vi "Drive Controller.vi"(8 "error in":errorcluster) -> ()   [LabVIEW 2017]
doc: "This VI executes continuously carrying out the current operation and responding to updates or new operation requests. It will often contain the timing or control code that is difficult to place directly in TeleOp. This VI generally opens all sensors and motors and isolates the rest of the robot code from knowing implementation details of how the operations are carried out."
uses:
  <vilib>/Rock Robotics/WPI/Framework/Completion Status.ctl
  Drive Setpoints.ctl
  Drive Operations.ctl
  <vilib>/Rock Robotics/WPI/SafetyOutput/WPI_SafetyOutputConfigMenu.ctl
  Public/Documents/Cross The Road Electronics/Phoenix-LabVIEW/Motor Controller/Controls/CTRE_Phoenix_MotorControl_FeedbackDevice.ctl
  Drive Published Globals.vi
  <vilib>/Rock Robotics/WPI/RobotDrive/WPI_RobotDriveOpen2MotorWithExistingMotors.vi
  Framework/Robot Global Data.vi
  Public/Documents/Cross The Road Electronics/Phoenix-LabVIEW/Motor Controller/Get/CTRE_Phoenix_MotorController_GetQuadratureData.vi
  <vilib>/Rock Robotics/WPI/RobotDrive/WPI_RobotDriveArcadeDrive_Standard(NoSaturation).vi
  <vilib>/Rock Robotics/Network Tables/NT Write Numeric Array.vi
panel:
  out "UseLDriveEncoder":bool
  out "LDriveEncoder":i32
  out "RDriveEncoder":i32
  out "DriveLastCommandStatus":T1
  in  "Interactive Values":T2
  in  "Buttons":cluster{"Execute Cmd":bool, "Abort Cmd":bool}
  out "Command Timing":cluster{"Start Time (ms)":u32, "Iterations":i32}
  out "Status":T1
  out "Setpoints":T4(graph)
  out "Current\nCmd":string
  # "Tip: The graph shows the motor setpoints. It may also be helpful to observe inputs and sensor values.\nYou may also want to display tuning or debugging controls."
  # "Interactive Command: You may fill in the settings for a command\nand schedule it with the Execute button. You can observe and abort\nany command while fine tuning the code for the controller."
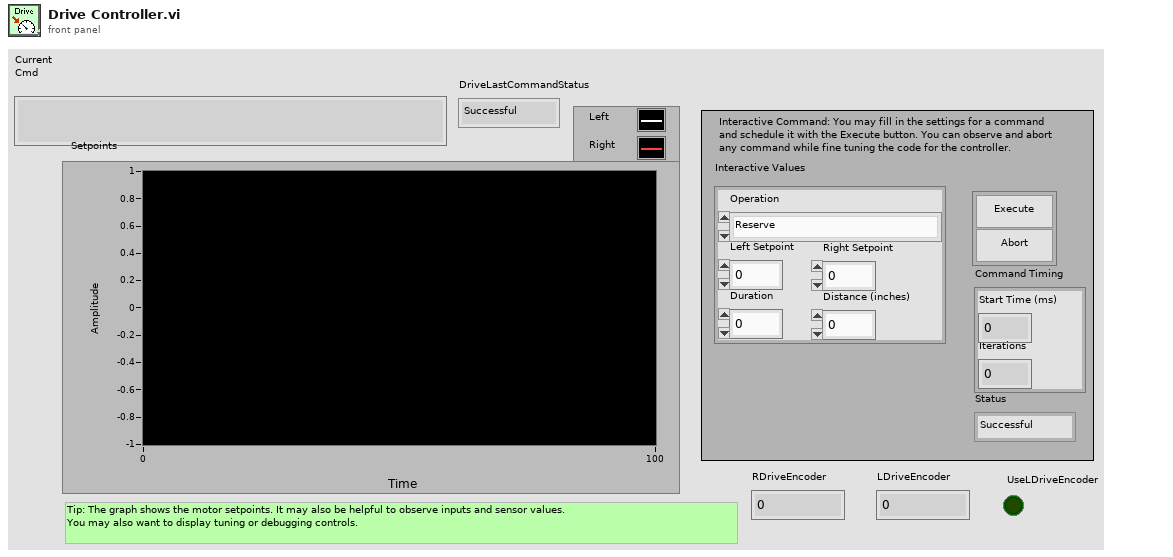
[diagram p1: front panel]
types:
  T1 = typedef "Completion Status.ctl" = enum16{"Successful", "Aborted", "Incomplete"}
  T2 = typedef "Drive Setpoints.ctl" = cluster{"Operation":T3, "Left Setpoint":dbl, "Right Setpoint":dbl, "Duration":dbl, "Distance (inches)":dbl}
  T3 = typedef "Drive Operations.ctl" = enum16{"Reserve", "Read Current", "Immediate", "Drive for Time", "Drive for Distance"}
  T4 = cluster{"Left Setpoint":dbl, "Right Setpoint":dbl}
  T5 = typedef "WPI_SafetyOutputConfigMenu.ctl" = enum16{"Enable", "Disable"}
  T6 = typedef "CTRE_Phoenix_MotorControl_FeedbackDevice.ctl" = i8
  T7 = typedef "WPI_MotorControlDeviceRef.ctl" = cluster{"DeviceStatus":errorcluster, "Type":T8, "PWM":cluster{"PWM Channel":T9, "DeadBand":T10}, "CAN":cluster{"Device Number":u8, "SetOutput VI Ref":variant, "GetOutput VI Ref":variant, "Enable VI Ref":variant, "Disable VI Ref":variant, "Data":variant}, "Invert":bool, "DIO PWM":cluster{"PWM \"Enable\" Channel":T9, "DIOChannel":T11, "PWM Rate":dbl}}
  T8 = typedef "WPI_MotorControlType.ctl" = enum16{"PWM", "CAN", "DIO PWM"}
  T9 = typedef "FPGA_DIOPWMChannel.ctl" = enum8{"PWM 0", "PWM 1", "PWM 2", "PWM 3", "PWM 4", "PWM 5", "PWM 6", "PWM 7", "PWM 8", "PWM 9", "PWM MXP 0", "PWM MXP 1", "PWM MXP 2", "PWM MXP 3", "PWM MXP 4", "PWM MXP 5", "PWM MXP 6", "PWM MXP 7", "PWM MXP 8", "PWM MXP 9", "Invalid"}
  T10 = typedef "WPI_PWMDeadband.ctl" = cluster{"Name":string, "maxPositivePwm":i32, "minPositivePwm":i32, "centerPwm":i32, "maxNegativePwm":i32, "minNegativePwm":i32, "angularRange":u16}
  T11 = typedef "FPGA_DIOChannel.ctl" = enum8{"DIO 0", "DIO 1", "DIO 2", "DIO 3", "DIO 4", "DIO 5", "DIO 6", "DIO 7", "DIO 8", "DIO 9", "DIO MXP 0", "DIO MXP 1", "DIO MXP 2", "DIO MXP 3", "DIO MXP 4", "DIO MXP 5", "DIO MXP 6", "DIO MXP 7", "DIO MXP 8", "DIO MXP 9", "DIO MXP 10", "DIO MXP 11", "DIO MXP 12", "DIO MXP 13", "DIO MXP 14", "DIO MXP 15", "SPI Port CS1", "SPI Port CS2", "SPI Port CS3", "SPI Port MISO", "SPI Port MOSI", "Invalid"}
  T12 = typedef "WPI_RobotDriveDevRef.ctl" = cluster{"DevStatus":errorcluster, "Motors[]":T7[], "Square Inputs":bool, "Max Output":dbl}
  T13 = typedef "Command Status Info.ctl" = cluster{"Name":string, "Status":T1, "notifier out":T14}
  T14 = typedef "Completion Notifier.ctl" = refnum<notifier>
  T15 = cluster{"SubSystem Data":T2, cluster{"Start Time (ms)":u32, "Iterations":i32}, cluster{"Command Info":T13, "Description":string, "Default Command":T2, "queue out":refnum<queue>, "Subsystem Name":string}}
  T16 = cluster{"SubSystem Data":T2, cluster{"Start Time (ms)":u32, "Iterations":i32}, "Default Command Arguments":cluster{"Command Info":T13, "Description":string, "Default Command":T2, "queue out":refnum<queue>, "Subsystem Name":string}}
  T17 = cluster{"Don't move motors while reserved":dbl, "Don't move motors while reserved":dbl}
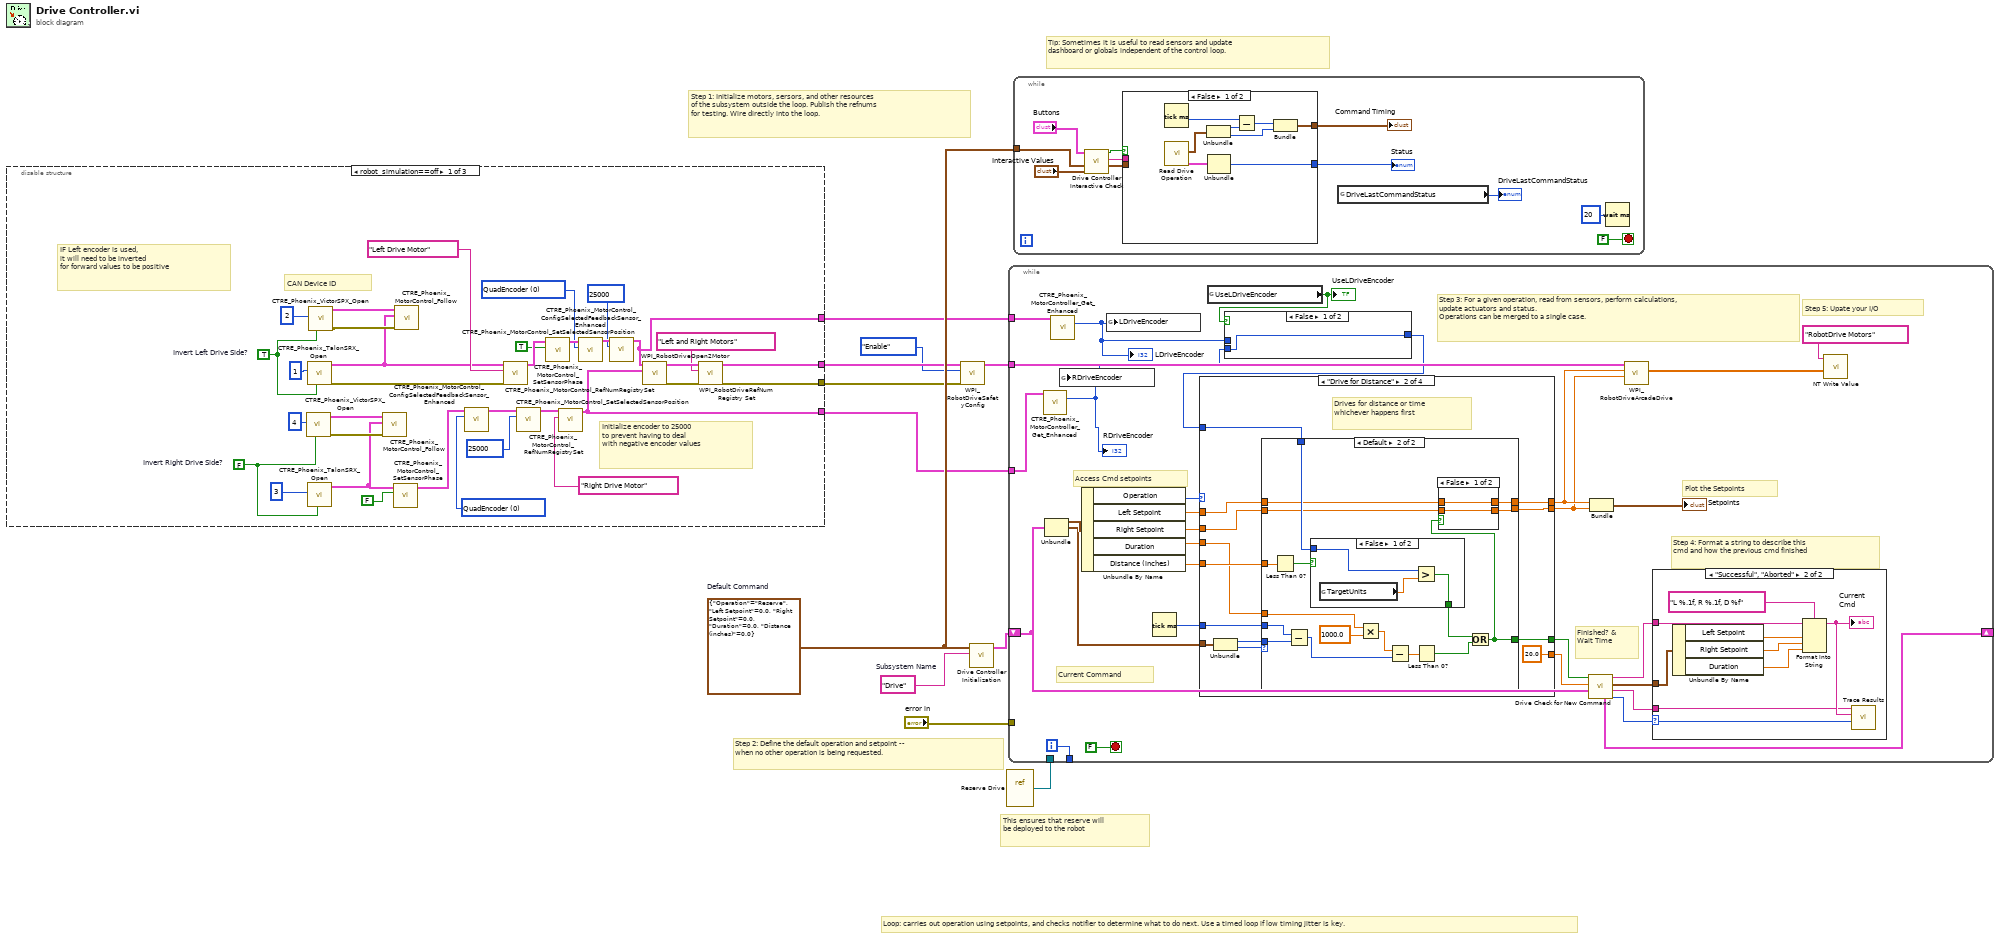
[diagram p0: block diagram]
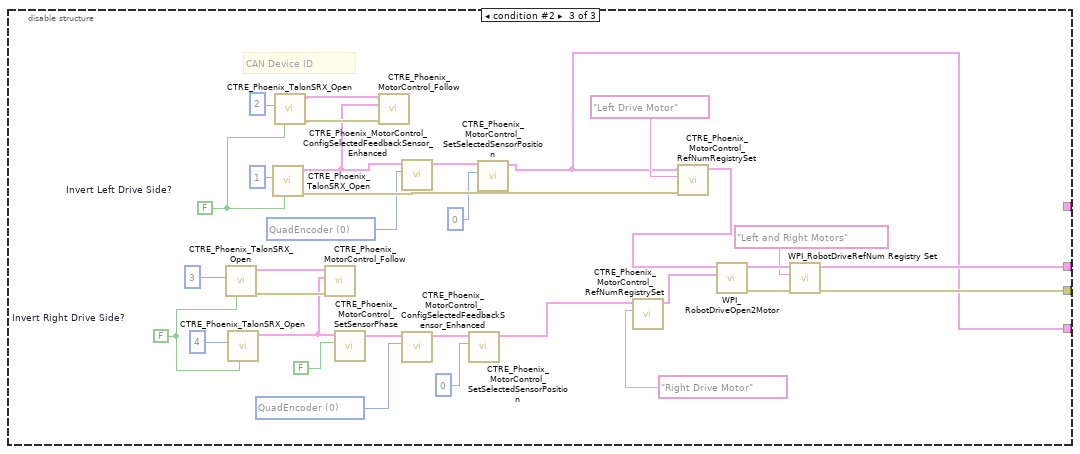
[diagram p3: hidden frame]
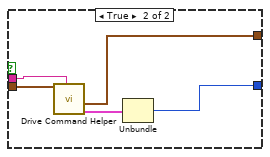
[diagram p4: hidden frame]
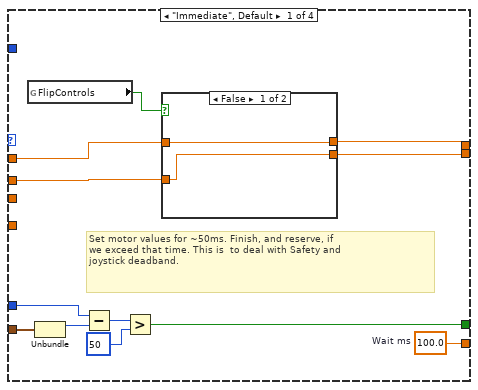
[diagram p7: hidden frame]
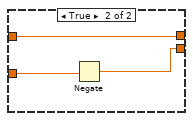
[diagram p8: hidden frame]
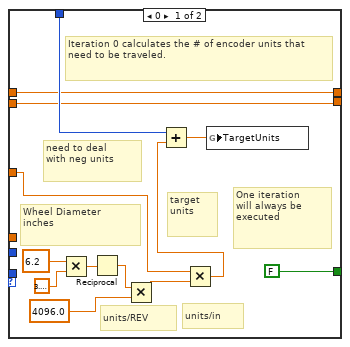
[diagram p9: hidden frame]
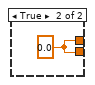
[diagram p10: hidden frame]
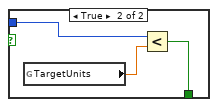
[diagram p11: hidden frame]
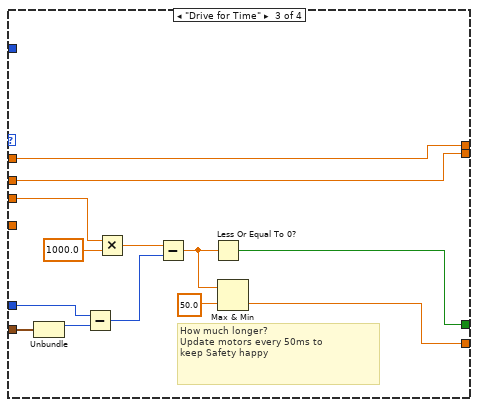
[diagram p12: hidden frame]
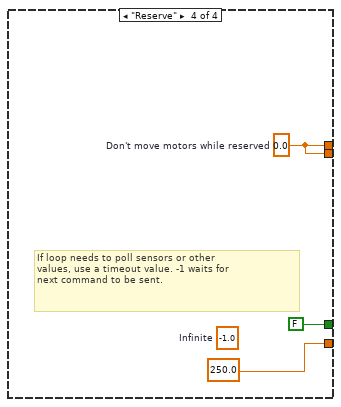
[diagram p13: hidden frame]
diagram:
  w6 = T2 {"Operation"=enum."Reserve", "Left Setpoint"=0.0, "Right Setpoint"=0.0, "Duration"=0.0, "Distance (inches)"=0.0}  # Default Command
  w11 = "Drive"  # Subsystem Name
  # "This ensures that reserve will\nbe deployed to the robot"
  # "Tip: Sometimes it is useful to read sensors and update\ndashboard or globals independent of the control loop."
  # "Step 2: Define the default operation and setpoint --\nwhen no other operation is being requested."
  # "Step 1: Initialize motors, sersors, and other resources\nof the subsystem outside the loop. Publish the refnums\nfor testing. Wire directly into the loop."
  # "Loop: carries out operation using setpoints, and checks notifier to determine what to do next. Use a timed loop if low timing jitter is key."
  n1 = disable-structure shown="robot_simulation==off" {
    disable-tunnel: [w38 _ w60] -> w5
    disable-tunnel: [w37 _ w59] -> w4
    disable-tunnel: [w19 _ w46] -> w2
    disable-tunnel: [w12 _ _] -> w1
    frame condition #0 (active) {
      w14 = T6 0 items=["None"=-1, "QuadEncoder"=0, "Analog"=2, "Tachometer"=4, "Pulse Width Encoded Position"=8, "Sensor Sum (S0 + S1)"=9, "Sensor Difference (D0 - D1)"=10, "Remote Source 0"=11, "Remote Source 1"=12, "Software Emulated"=15] ("Feedback Device")
      w24 = T6 0 items=["None"=-1, "QuadEncoder"=0, "Analog"=2, "Tachometer"=4, "Pulse Width Encoded Position"=8, "Sensor Sum (S0 + S1)"=9, "Sensor Difference (D0 - D1)"=10, "Remote Source 0"=11, "Remote Source 1"=12, "Software Emulated"=15] ("Feedback Device")
      w30 = TRUE  # Invert Left Drive Side?
      w28 = FALSE  # Invert Right Drive Side?
      # "IF Left encoder is used,\nit will need to be inverted\nfor forward values to be positive"
      # "Initialize encoder to 25000\nto prevent having to deal\nwith negative encoder values"
      # "CAN Device ID"
      n2 = call "CTRE_Phoenix_VictorSPX_Open.vi"("Invert"=w28, "Device Number"=u8 4) -> ("error out"=w40:errorcluster, "CAN Talon SRX Ref"=w39:T7)  [unwired: 8 in]
      n3 = call "CTRE_Phoenix_TalonSRX_Open.vi"("Invert"=w30, "Device Number"=u8 1) -> ("error out"=w41:errorcluster, "CAN Talon SRX Ref"=w31:T7)  [unwired: 8 in]
      n4 = call "CTRE_Phoenix_TalonSRX_Open.vi"("Invert"=w28, "Device Number"=u8 3) -> ("CAN Talon SRX Ref"=w26:T7)  [unwired: 8 in, 1 out]
      n5 = call "CTRE_Phoenix_VictorSPX_Open.vi"("Invert"=w30, "Device Number"=u8 2) -> ("error out"=w34:errorcluster, "CAN Talon SRX Ref"=w35:T7)  [unwired: 8 in]
      n6 = call "CTRE_Phoenix_MotorControl_Follow.vi"("error in (no error)"=w40, "Master Controller to Follow"=w26, "PhoenixMotorControlDevRef"=w39) -> ()  [unwired: 7 in, 2 out]
      n7 = call "CTRE_Phoenix_MotorControl_SetSensorPhase.vi"("PhaseSensor"=FALSE, "PhoenixMotorControlDevRef"=w26) -> ("PhoenixMotorControlDevRef"=w22:T7)  [unwired: 8 in, 1 out]
      n8 = call "CTRE_Phoenix_MotorControl_Follow.vi"("error in (no error)"=w34, "Master Controller to Follow"=w31, "PhoenixMotorControlDevRef"=w35) -> ()  [unwired: 7 in, 2 out]
      n9 = call "CTRE_Phoenix_MotorControl_ConfigSelectedFeedbackSensor_Enhanced.vi"("Feedback Device"=w24, "PhoenixMotorControlDevRef"=w22) -> ("PhoenixMotorControlDevRef"=w21:T7)  [unwired: 8 in, 1 out]
      n10 = call "CTRE_Phoenix_MotorControl_RefNumRegistrySet.vi"("error in (no error)"=w41, "refnum name"="Left Drive Motor", "PhoenixMotorControlDevRef"=w31) -> ("PhoenixMotorControlDevRef"=w17:T7)  [unwired: 7 in, 1 out]
      n11 = call "CTRE_Phoenix_MotorControl_SetSelectedSensorPosition.vi"("New Sensor Position"=25000, "PhoenixMotorControlDevRef"=w21) -> ("PhoenixMotorControlDevRef"=w20:T7)  [unwired: 8 in, 1 out]
      n12 = call "CTRE_Phoenix_MotorControl_SetSensorPhase.vi"("PhaseSensor"=TRUE, "PhoenixMotorControlDevRef"=w17) -> ("PhoenixMotorControlDevRef"=w16:T7)  [unwired: 8 in, 1 out]
      n13 = call "CTRE_Phoenix_MotorControl_RefNumRegistrySet.vi"("refnum name"="Right Drive Motor", "PhoenixMotorControlDevRef"=w20) -> ("PhoenixMotorControlDevRef"=w19:T7)  [unwired: 8 in, 1 out]
      n14 = call "CTRE_Phoenix_MotorControl_ConfigSelectedFeedbackSensor_Enhanced.vi"("Feedback Device"=w14, "PhoenixMotorControlDevRef"=w16) -> ("PhoenixMotorControlDevRef"=w18:T7)  [unwired: 8 in, 1 out]
      n15 = call "CTRE_Phoenix_MotorControl_SetSelectedSensorPosition.vi"("New Sensor Position"=25000, "PhoenixMotorControlDevRef"=w18) -> ("PhoenixMotorControlDevRef"=w12:T7)  [unwired: 8 in, 1 out]
      n16 = call-poly <vilib>:"WPI_RobotDriveOpen2Motor.vi"("Right Motor Dev Ref"=w19, "Left Motor Dev Ref"=w12) -> ("error out"=w43:errorcluster, "RobotDriveDevRef"=w45:T12)  [unwired: 3 in, 5 out]
      n17 = call <vilib>:"WPI_RobotDriveRefNum Registry Set.vi"("error in (no error)"=w43, "refnum name"="Left and Right Motors", "RobotDriveDevRef"=w45) -> ("error out"=w37:errorcluster, "RobotDriveDevRef"=w38:T12)  [unwired: 1 in, 6 out]
    }
    frame condition #1 {
    }
    frame condition #2 {
      w47 = T6 0 items=["None"=-1, "QuadEncoder"=0, "Analog"=2, "Tachometer"=4, "Pulse Width Encoded Position"=8, "Sensor Sum (S0 + S1)"=9, "Sensor Difference (D0 - D1)"=10, "Remote Source 0"=11, "Remote Source 1"=12, "Software Emulated"=15] ("Feedback Device")
      w52 = T6 0 items=["None"=-1, "QuadEncoder"=0, "Analog"=2, "Tachometer"=4, "Pulse Width Encoded Position"=8, "Sensor Sum (S0 + S1)"=9, "Sensor Difference (D0 - D1)"=10, "Remote Source 0"=11, "Remote Source 1"=12, "Software Emulated"=15] ("Feedback Device")
      w67 = FALSE  # Invert Left Drive Side?
      w58 = FALSE  # Invert Right Drive Side?
      # "CAN Device ID"
      n18 = call "CTRE_Phoenix_TalonSRX_Open.vi"("Invert"=w58, "Device Number"=u8 3) -> ("error out"=w70:errorcluster, "CAN Talon SRX Ref"=w69:T7)  [unwired: 8 in]
      n19 = call "CTRE_Phoenix_TalonSRX_Open.vi"("Invert"=w58, "Device Number"=u8 4) -> ("CAN Talon SRX Ref"=w57:T7)  [unwired: 8 in, 1 out]
      n20 = call "CTRE_Phoenix_TalonSRX_Open.vi"("Invert"=w67, "Device Number"=u8 1) -> ("error out"=w72:errorcluster, "CAN Talon SRX Ref"=w50:T7)  [unwired: 8 in]
      n21 = call "CTRE_Phoenix_TalonSRX_Open.vi"("Invert"=w67, "Device Number"=u8 2) -> ("error out"=w64:errorcluster, "CAN Talon SRX Ref"=w65:T7)  [unwired: 8 in]
      n22 = call "CTRE_Phoenix_MotorControl_Follow.vi"("error in (no error)"=w70, "Master Controller to Follow"=w57, "PhoenixMotorControlDevRef"=w69) -> ()  [unwired: 7 in, 2 out]
      n23 = call "CTRE_Phoenix_MotorControl_SetSensorPhase.vi"("PhaseSensor"=FALSE, "PhoenixMotorControlDevRef"=w57) -> ("PhoenixMotorControlDevRef"=w54:T7)  [unwired: 8 in, 1 out]
      n24 = call "CTRE_Phoenix_MotorControl_Follow.vi"("error in (no error)"=w64, "Master Controller to Follow"=w50, "PhoenixMotorControlDevRef"=w65) -> ()  [unwired: 7 in, 2 out]
      n25 = call "CTRE_Phoenix_MotorControl_ConfigSelectedFeedbackSensor_Enhanced.vi"("Feedback Device"=w47, "PhoenixMotorControlDevRef"=w50) -> ("PhoenixMotorControlDevRef"=w49:T7)  [unwired: 8 in, 1 out]
      n26 = call "CTRE_Phoenix_MotorControl_ConfigSelectedFeedbackSensor_Enhanced.vi"("Feedback Device"=w52, "PhoenixMotorControlDevRef"=w54) -> ("PhoenixMotorControlDevRef"=w55:T7)  [unwired: 8 in, 1 out]
      n27 = call "CTRE_Phoenix_MotorControl_SetSelectedSensorPosition.vi"("New Sensor Position"=0, "PhoenixMotorControlDevRef"=w55) -> ("PhoenixMotorControlDevRef"=w51:T7)  [unwired: 8 in, 1 out]
      n28 = call "CTRE_Phoenix_MotorControl_SetSelectedSensorPosition.vi"("New Sensor Position"=0, "PhoenixMotorControlDevRef"=w49) -> ("PhoenixMotorControlDevRef"=w46:T7)  [unwired: 8 in, 1 out]
      n29 = call "CTRE_Phoenix_MotorControl_RefNumRegistrySet.vi"("refnum name"="Right Drive Motor", "PhoenixMotorControlDevRef"=w51) -> ("PhoenixMotorControlDevRef"=w62:T7)  [unwired: 8 in, 1 out]
      n30 = call "CTRE_Phoenix_MotorControl_RefNumRegistrySet.vi"("error in (no error)"=w72, "refnum name"="Left Drive Motor", "PhoenixMotorControlDevRef"=w46) -> ("PhoenixMotorControlDevRef"=w61:T7)  [unwired: 7 in, 1 out]
      n31 = call-poly <vilib>:"WPI_RobotDriveOpen2Motor.vi"("Right Motor Dev Ref"=w62, "Left Motor Dev Ref"=w61) -> ("error out"=w75:errorcluster, "RobotDriveDevRef"=w77:T12)  [unwired: 3 in, 5 out]
      n32 = call <vilib>:"WPI_RobotDriveRefNum Registry Set.vi"("error in (no error)"=w75, "refnum name"="Left and Right Motors", "RobotDriveDevRef"=w77) -> ("error out"=w59:errorcluster, "RobotDriveDevRef"=w60:T12)  [unwired: 1 in, 6 out]
    }
  }
  n33 = call <vilib>:"WPI_RobotDriveSafetyConfig.vi"("error in (no error)"=w4, "mode"=WPI_SafetyOutputConfigMenu."Enable", "RobotDriveDevRef"=w5) -> ("RobotDriveDevRef"=w10:T12)  [unwired: 7 in, 1 out]
  n34 = call "Drive Controller Initialization.vi"("Subsystem Name"=w11, "Default Command"=w6) -> ("Current Command"=w8:T15)  [unwired: 9 in]
  n35 = vi-ref "Reserve Drive.vi"() -> (w7:refnum<vi>)
  n36 = while {
    shift-right: [w95] -> _
    shift-left: w8 -> [w88]
    tunnel: [w106] -> _
    tunnel: w10 -> [w84]
    tunnel: "error in" -> [_]
    tunnel: w7 -> [_]
    tunnel: w2 -> [w83]
    tunnel: w1 -> [w82]
    i -> [w106]
    stop <- FALSE stop-if-true
    # "Step 5: Upate your I/O"
    # "Step 4: Format a string to describe this\ncmd and how the previous cmd finished"
    # "Current Command"
    # "Plot the Setpoints"
    # "Access Cmd setpoints"
    # "Finished? &\nWait Time"
    # "Step 3: For a given operation, read from sensors, perform calculations,\nupdate actuators and status.\nOperations can be merged to a single case."
    n37 = call-poly "CTRE_Phoenix_MotorController_Get_Enhanced.vi"("PhoenixMotorControlDevRef"=w83) -> ("Quadrature Position"=w80:i32)  [unwired: 11 in, 3 out]
    "RDriveEncoder" <- w80
    n38 = Unbundle(w88) -> ("SubSystem Data"=w102:T2, w89:cluster{"Start Time (ms)":u32, "Iterations":i32})  [unwired: 1 out]
    n39 = call-poly "CTRE_Phoenix_MotorController_Get_Enhanced.vi"("PhoenixMotorControlDevRef"=w82) -> ("Quadrature Position"=w81:i32)  [unwired: 11 in, 3 out]
    "LDriveEncoder" <- w81
    n40 = global write "Robot Global Data.vi" "RDriveEncoder"(w80) -> ()
    n41 = Unbundle By Name(w102) -> ("Operation"=w101:T3, "Left Setpoint"=w100:dbl, "Right Setpoint"=w99:dbl, "Duration"=w98:dbl, "Distance (inches)"=w85:dbl)
    n42 = global write "Robot Global Data.vi" "LDriveEncoder"(w81) -> ()
    n43 = Tick Count (ms)() -> (millisecond timer value=w97:u32)
    n44 = global read "Robot Global Data.vi" "UseLDriveEncoder"() -> (w78:bool)
    "UseLDriveEncoder" <- w78
    n45 = case shown="False" w78 {
      tunnel: [w108 w109] -> w79
      tunnel: w81 -> [_ w109]
      tunnel: w80 -> [w108 _]
      frame False {
      }
      frame True {
      }
    }
    n46 = case shown="\"Drive for Distance\"" w101 {
      tunnel: [w130 20.0 ("Infinite") w188 250.0 ("Infinite")] -> w94
      tunnel: [w125 w145 w195 FALSE ("ignore previous (F)")] -> w93
      tunnel: w89 -> [w124 w148 w197 _]
      tunnel: [w121 w140 w194 w202] -> w104
      tunnel: [w120 w139 w193 w202] -> w103
      tunnel: w100 -> [w123 w137 w194 _]
      tunnel: w99 -> [w122 w138 w193 _]
      tunnel: w98 -> [_ w141 w192 _]
      tunnel: w97 -> [w126 w142 w191 _]
      tunnel: w85 -> [_ w146 _ _]
      tunnel: w79 -> [_ w136 _ _]
      frame "Immediate", Default {
        w130 = 100.0  # Wait ms
        # "Set motor values for ~50ms. Finish, and reserve, if\nwe exceed that time. This is  to deal with Safety and\njoystick deadband."
        n47 = global read "Robot Global Data.vi" "FlipControls"() -> (w119:bool)
        n48 = Unbundle(w124) -> ("Start Time (ms)"=w127:u32)  [unwired: 1 out]
        n49 = Subtract(x=w126, y=w127) -> (x-y=w128:u32)
        n50 = Greater?(x=w128, y=u8 50 ("Left Motor")) -> (0:w125:bool)
        n51 = case shown="False" w119 {
          tunnel: w123 -> [w132 w133]
          tunnel: w122 -> [w131 w135]
          tunnel: [w132 w133] -> w121
          tunnel: [w131 w134] -> w120
          frame False {
          }
          frame True {
            n52 = Negate(x=w135) -> (-x=w134:dbl)
          }
        }
      }
      frame "Drive for Distance" {
        # "Drives for distance or time\nwhichever happens first"
        n53 = Unbundle(w148) -> ("Start Time (ms)"=w143:u32, "Iterations"=w147:i32)
        n54 = case shown="Default" w147 {
          tunnel: w146 -> [w159 w178]
          tunnel: w136 -> [w154 w176]
          tunnel: [FALSE w162] -> w145
          tunnel: w143 -> [_ w175]
          tunnel: w142 -> [_ w174]
          tunnel: w141 -> [_ w172]
          tunnel: [w150 w166] -> w140
          tunnel: w138 -> [w149 w164]
          tunnel: [w149 w163] -> w139
          tunnel: w137 -> [w150 w165]
          frame 0 {
            # "need to deal\nwith neg units"
            # "One iteration\nwill always be\nexecuted"
            # "Iteration 0 calculates the # of encoder units that need to be traveled."
            # "target\nunits"
            # "units/in"
            # "units/REV"
            # "Wheel Diameter \ninches"
            n55 = Multiply(x=6.2, y=3.141592653589793) -> (x*y=w157:dbl)
            n56 = Reciprocal(x=w157) -> (1/x=w156:dbl)
            n57 = Multiply(x=w156, y=4096.0 ("x")) -> (x*y=w158:dbl)
            n58 = Multiply(x=w159, y=w158) -> (x*y=w153:dbl)
            n59 = Add(x=w154, y=w153) -> (x+y=w152:dbl)
            n60 = global write "Drive Published Globals.vi" "TargetUnits"(w152) -> ()
          }
          frame Default {
            n61 = Less Than 0?(x=w178) -> (x < 0?=w177:bool)
            n62 = Subtract(x=w174, y=w175) -> (x-y=w170:u32)
            n63 = case shown="False" w177 {
              tunnel: w176 -> [w183 w186]
              tunnel: [w182 w185] -> w168
              frame False {
                n64 = global read "Drive Published Globals.vi" "TargetUnits"() -> (w184:dbl)
                n65 = Greater?(x=w183, y=w184) -> (0:w182:bool)
              }
              frame True {
                n66 = global read "Drive Published Globals.vi" "TargetUnits"() -> (w187:dbl)
                n67 = Less?(x=w186, y=w187) -> (x < y?=w185:bool)
              }
            }
            n68 = Multiply(x=w172, y=1000.0) -> (x*y=w171:dbl)
            n69 = Subtract(x=w171, y=w170) -> (x-y=w169:dbl)
            n70 = Less Than 0?(x=w169) -> (x < 0?=w167:bool)
            n71 = Or(x=w168, y=w167) -> (x .or. y?=w162:bool)
            n72 = case shown="False" w162 {
              tunnel: [w180 w181] -> w166
              tunnel: w165 -> [w180 _]
              tunnel: w164 -> [w179 _]
              tunnel: [w179 w181] -> w163
              frame False {
              }
              frame True {
                w181 = 0.0 ("Left Setpoint")
              }
            }
          }
        }
      }
      frame "Drive for Time" {
        # "How much longer?\nUpdate motors every 50ms to\nkeep Safety happy"
        n73 = Unbundle(w197) -> ("Start Time (ms)"=w196:u32)  [unwired: 1 out]
        n74 = Subtract(x=w191, y=w196) -> (x-y=w200:u32)
        n75 = Multiply(x=w192, y=1000.0) -> (x*y=w199:dbl)
        n76 = Subtract(x=w199, y=w200) -> (x-y=w190:dbl)
        n77 = Less Or Equal To 0?(x=w190) -> (x <= 0?=w195:bool)
        n78 = Max & Min(x=w190, y=50.0) -> (min(x,y)=w188:dbl)  [unwired: 1 out]
      }
      frame "Reserve" {
        w202 = 0.0  # Don't move motors while reserved
        (unwired) -1.0  # Infinite
        # "If loop needs to poll sensors or other\nvalues, use a timeout value. -1 waits for\nnext command to be sent."
      }
    }
    n79 = call "Drive Check for New Command.vi"("input cluster"=w88, "Wait time (ms)"=w94, "Finished?"=w93) -> ("Completion"=w96:T1, "Subsystem Name"=w90:string, "Current Command"=w91:T2, "Initial Trace String"=w92:string, "Next Command"=w95:T16)  [unwired: 4 in]
    n80 = Bundle("Don't move motors while reserved"=w104, "Don't move motors while reserved"=w103) -> (→"Setpoints":T17)  [unwired: 1 in]
    n81 = call-poly <vilib>:"WPI_RobotDriveArcadeDrive.vi"("Y axis value"=w103, "X axis value"=w104, "RobotDriveDevRef"=w84) -> ("Motor Values"=w86:dbl[])  [unwired: 6 in, 2 out]
    n82 = case shown="\"Successful\", \"Aborted\"" w96 {
      selector: w96 -> [_ w118]
      tunnel: w92 -> [_ w113]
      tunnel: w91 -> [_ w114]
      tunnel: w90 -> [_ w110]
      frame "Incomplete", Default {
        # "Continuing current command"
      }
      frame "Successful", "Aborted" {
        # "Report and setup for next command"
        n83 = Unbundle By Name(w114) -> ("Left Setpoint"=w116:dbl, "Right Setpoint"=w117:dbl, "Duration"=w111:dbl)
        n84 = Format Into String(format string="L %.1f, R %.1f, D %f", initial string=w113, w116, w117, w111) -> (resulting string=w112:string)  [unwired: 1 in, 1 out]
        "Current\nCmd" <- w112
        n85 = call <vilib>:"Trace Results.vi"("Status of previous command"=w118, "Description"=w112, "Subsystem"=w110) -> ()  [unwired: 9 in]
      }
    }
    n86 = call-poly <vilib>:"NT Write Value.vi"("Numeric Array"=w86, "Name"="RobotDrive Motors") -> ()  [unwired: 9 in, 1 out]
  }
  n87 = while {
    tunnel: w6 -> [w206]
    stop <- FALSE stop-if-true
    n88 = call "Drive Controller Interactive Check.vi"("Interactive Command In"="Interactive Values", "Default Command"=w206, "Buttons"="Buttons") -> ("Interactive Command Out"=w208:T2, "Trace String"=w209:string, "Schedule"=w210:bool)  [unwired: 6 in]
    n89 = case shown="False" w210 {
      tunnel: [w219 w227] -> w211
      tunnel: [w218 w223] -> w212
      tunnel: w209 -> [_ w225]
      tunnel: w208 -> [_ w224]
      frame False {
        n90 = Tick Count (ms)() -> (millisecond timer value=w222:u32)
        n91 = call "Read Drive Operation.vi"() -> ("Command Info"=w216:T13, "Command Timing"=w215:cluster{"Start Time (ms)":u32, "Iterations":i32})  [unwired: 9 in, 1 out]
        n92 = Unbundle(w215) -> ("Start Time (ms)"=w220:u32, "Iterations"=w217:i32)
        n93 = Unbundle(w216) -> ("Status"=w219:T1)  [unwired: 2 out]
        n94 = Subtract(x=w222, y=w220) -> (x-y=w221:u32)
        n95 = Bundle(w221, "Iterations"=w217) -> (w218:cluster{u32, "Iterations":i32})  [unwired: 1 in]
      }
      frame True {
        n96 = call "Drive Command Helper.vi"("Description"=w225, "SubSystem Data"=w224) -> ("Command Info Out"=w226:T13, "Command Timing"=w223:cluster{"Start Time (ms)":u32, "Iterations":i32})  [unwired: 7 in, 1 out]
        n97 = Unbundle(w226) -> ("Status"=w227:T1)  [unwired: 2 out]
      }
    }
    "Status" <- w211
    "Command Timing" <- w212
    n98 = global read "Drive Published Globals.vi" "DriveLastCommandStatus"() -> (→"DriveLastCommandStatus":T1)
    n99 = Wait (ms)(milliseconds to wait=u32 20) -> ()  [unwired: 1 out]
  }
